vi "VG_Conti.vi"() -> ()   [LabVIEW 2020]
panel:
  out "Conti":dbl
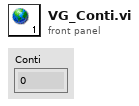
[diagram p1: front panel]
diagram:
